vi "Stop.vi"(8 "error in (no error)":errorcluster, 10 "Message in":refnum<class "StopMessage.lvclass">, 11 "DAQMH121119OrcaFlash in":refnum<class "DAQOrcaFlash.lvclass">) -> (0 "error out":errorcluster, 3 "DAQMH121119OrcaFlash out":refnum<class "DAQOrcaFlash.lvclass">)   [LabVIEW 2012, in "DAQOrcaFlash.lvclass"]
doc: "This member function is called when the statemachine in the run.vi receives an 'stop' command. It relays the message to all observers of the component.\n\nOverride this member function in your derived class if you need additional stop functionality (but don't forget to call the parent method)."
uses:
  DAQOrcaFlash.lvclass
  <vilib>/Distrio/Murmex/StopMessage/StopMessage.lvclass
  <vilib>/Distrio/Murmex/Murmex/Murmex.lvclass
  DAQOrcaFlash.lvclass/DAQOrcaFlash.ctl
  imaging_mode.ctl
panel:
  # "This method is called when the STOP\ntrigger is sent. \n\nOverride this method when your component needs to\nrespond to this trigger. \n\nCall parent for proper implementation"
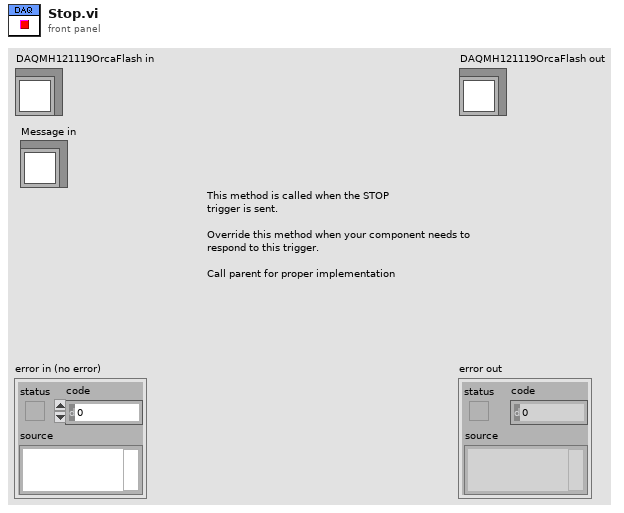
[diagram p1: front panel]
types:
  T1 = typedef "DAQOrcaFlash.lvclass/imaging_mode.ctl" = enum16{"focus mode", "single sweep"}
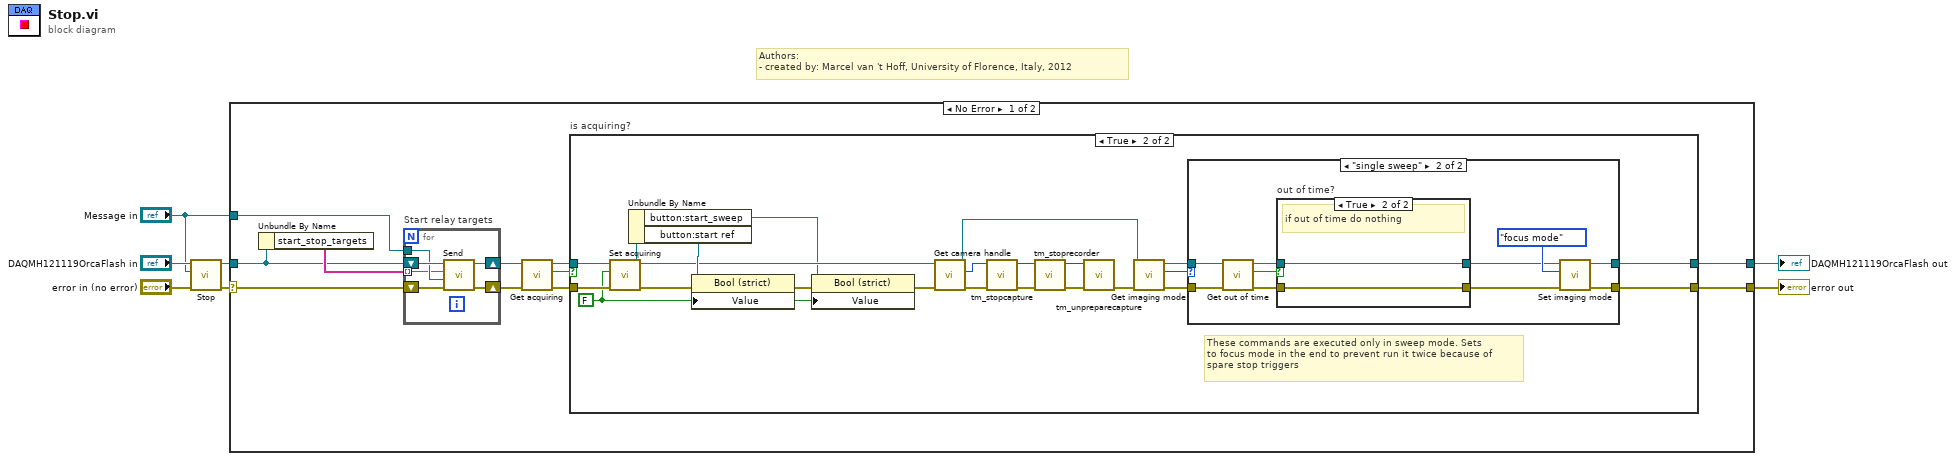
[diagram p0: block diagram]
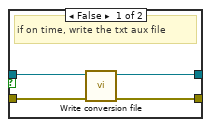
[diagram p4: hidden frame]
diagram:
  # "Authors: \n- created by: Marcel van 't Hoff, University of Florence, Italy, 2012"
  n1 = call-parent "Stop.vi"("error in (no error)"="error in (no error)", "Message in"="Message in", "Murmex in"="DAQMH121119OrcaFlash in") -> ("error out"=w5:errorcluster, "Murmex out"=w2:refnum<class "DAQOrcaFlash.lvclass">)  [unwired: 7 in]
  n2 = case shown="No Error" w5 {
    selector: w5 -> [w14 w67]
    tunnel: [w9 w67] -> w4
    tunnel: [w8 w68] -> w3
    tunnel: w2 -> [w12 w68]
    tunnel: "Message in" -> [w10 _]
    frame No Error {
      n3 = Unbundle By Name(w12) -> ("start_stop_targets"=w15:string[])
      n4 = for "Start relay targets" {
        shift-right: [w24] -> w13
        shift-left: w14 -> [w23]
        tunnel: w10 -> [w21]
        tunnel: w15 -> [w20] mode=indexing
        shift-right: [w19] -> w11
        shift-left: w12 -> [w22]
        n5 = call <vilib>:"Send.vi"("error in (no error)"=w23, "Message"=w21, "recipient"=w20, "Murmex in"=w22) -> ("error out"=w24:errorcluster, "Murmex out"=w19:refnum<class "DAQOrcaFlash.lvclass">)  [unwired: 6 in]
      }
      n6 = call "Get acquiring.vi"("error in (no error)"=w13, "DAQMH121119OrcaFlash in"=w11) -> ("error out"=w17:errorcluster, "is acquiring?"=w16:bool, "DAQMH121119OrcaFlash out"=w18:refnum<class "DAQOrcaFlash.lvclass">)  [unwired: 7 in]
      n7 = case "is acquiring?" shown="True" w16 {
        tunnel: [w25 w37] -> w8
        tunnel: [w26 w38] -> w9
        tunnel: w18 -> [w25 w45]
        tunnel: w17 -> [w26 w44]
        frame False {
        }
        frame True {
          w40 = FALSE ("is acquiring?")
          # "These commands are executed only in sweep mode. Sets\nto focus mode in the end to prevent run it twice because of \nspare stop triggers"
          n8 = call "Set acquiring.vi"("error in (no error)"=w44, "is acquiring?"=w40, "DAQMH121119OrcaFlash in"=w45) -> ("error out"=w47:errorcluster, "DAQMH121119OrcaFlash out"=w46:refnum<class "DAQOrcaFlash.lvclass">)  [unwired: 7 in]
          n9 = Unbundle By Name(w46) -> ("button:start_sweep"=w43:refnum<vi>, "button:start ref"=w48:refnum<vi>)
          n10 = property class="Bool (strict)"(reference=w48, error in=w47, "Value"=w40) -> (error out=w42:errorcluster)  [unwired: 1 out]
          n11 = property class="Bool (strict)"(reference=w43, error in=w42, "Value"=w40) -> (error out=w41:errorcluster)  [unwired: 1 out]
          n12 = call "Get camera handle.vi"("error in (no error)"=w41, "DAQMH121119OrcaFlash in"=w46) -> ("error out"=w30:errorcluster, "cam handle"=w29:u32, "DAQMH121119OrcaFlash out"=w35:refnum<class "DAQOrcaFlash.lvclass">)  [unwired: 7 in]
          n13 = call <userlib>:"tm_stopcapture.vi"("error in (no error)"=w30, "Handle in"=w29) -> ("error out"=w31:errorcluster, "Handle out"=w28:u32)  [unwired: 8 in]
          n14 = call <userlib>:"tm_stoprecorder.vi"("error in (no error)"=w31, "Handle in"=w28) -> ("error out"=w32:errorcluster, "Handle out"=w27:u32)  [unwired: 8 in]
          n15 = call <userlib>:"tm_unpreparecapture.vi"("error in (no error)"=w32, "Handle in"=w27) -> ("error out"=w39:errorcluster)  [unwired: 8 in, 1 out]
          n16 = call "Get imaging mode.vi"("error in (no error)"=w39, "DAQMH121119OrcaFlash in"=w35) -> ("error out"=w36:errorcluster, "imaging mode"=w33:T1, "DAQMH121119OrcaFlash out"=w34:refnum<class "DAQOrcaFlash.lvclass">)  [unwired: 7 in]
          n17 = case shown="\"single sweep\"" w33 {
            tunnel: w36 -> [w49 w55]
            tunnel: [w49 w60] -> w38
            tunnel: [w50 w59] -> w37
            tunnel: w34 -> [w50 w54]
            frame "focus mode", Default {
            }
            frame "single sweep" {
              n18 = call-dynamic "Get out of time.vi"("error in (no error)"=w55, "DAQOrcaFlash in"=w54) -> ("error out"=w51:errorcluster, "out of time?"=w53:bool, "DAQOrcaFlash out"=w52:refnum<class "DAQOrcaFlash.lvclass">)  [unwired: 7 in]
              n19 = case "out of time?" shown="True" w53 {
                tunnel: w51 -> [w64 w65]
                tunnel: [w63 w65] -> w57
                tunnel: w52 -> [w62 w66]
                tunnel: [w61 w66] -> w56
                frame False {
                  # "if on time, write the txt aux file"
                  n20 = call-dynamic "Write conversion file.vi"("error in (no error)"=w64, "DAQOrcaFlash in"=w62) -> ("error out"=w63:errorcluster, "DAQOrcaFlash out"=w61:refnum<class "DAQOrcaFlash.lvclass">)  [unwired: 8 in]
                }
                frame True {
                  # "if out of time do nothing"
                }
              }
              n21 = call "Set imaging mode.vi"("error in (no error)"=w57, "imaging mode"=imaging_mode."focus mode", "DAQMH121119OrcaFlash in"=w56) -> ("error out"=w60:errorcluster, "DAQMH121119OrcaFlash out"=w59:refnum<class "DAQOrcaFlash.lvclass">)  [unwired: 7 in]
            }
          }
        }
      }
    }
    frame Error {
    }
  }
  "error out" <- w4
  "DAQMH121119OrcaFlash out" <- w3
